vi "Slice Average calc.vi"(9 "end time (unix,ns)":u64, 10 "start time (unix,ns)":u64, 11 "Plot (unix)":T2) -> (2 "slice average":T1, 3 "Plot (unix)":T2)   [LabVIEW 2021, in "RocketPlot.lvlib"]
uses:
  RocketPlot.lvlib
  TypeDefs/plot datapoint.ctl
  TypeDefs/Slice average.ctl
  aeb3b9b0-3d0b-48fb-8ca9-3c9e8c208765.vi
  43998882-4a9d-44ca-a800-b6f182c48d79.vi
  <userlib>/bjustice/Ring Buffer for Time Series Data Strict Accessor/SubVIs/Search for oldest time to keep.vi
  <userlib>/bjustice/Ring Buffer for Time Series Data Strict Accessor/SubVIs/Search for newest time to keep.vi
  <userlib>/bjustice/Ring Buffer for Time Series Data Strict Accessor/Unix time epoch/Unix_Epoch_in_Labview.vi
  <vilib>/Analysis/NI_AALBase.lvlib
  <vilib>/Analysis/NI_AALPro.lvlib
  <userlib>/bjustice/Ring Buffer for Time Series Data Strict Accessor/Ring Buffer Strict Accessor.lvlib
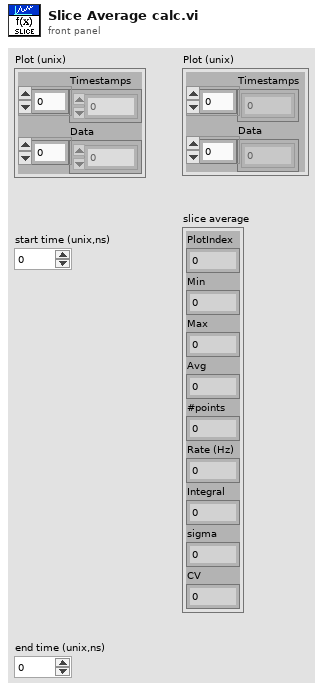
[diagram p1: front panel]
types:
  T1 = typedef "RocketPlot.lvlib/Slice average.ctl" = cluster{"PlotIndex":i32, "Min":dbl, "Max":dbl, "Avg":dbl, "#points":u32, "Rate (Hz)":dbl, "Integral":dbl, "sigma":dbl, "CV":dbl}
  T2 = typedef "RocketPlot.lvlib/plot datapoint.ctl" = cluster{"Timestamps":u64[], "Data":dbl[]}
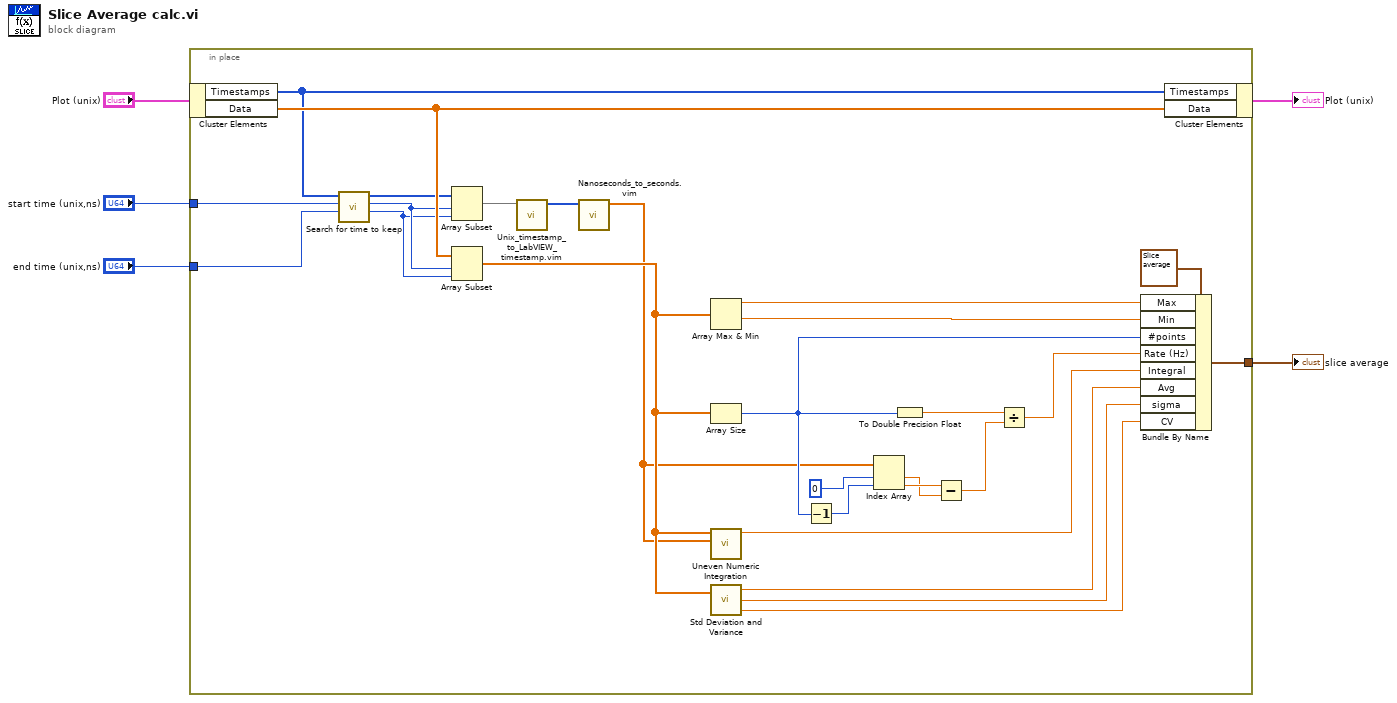
[diagram p0: block diagram]
diagram:
  n1 = in-place {
    in-place-border: "start time (unix,ns)" -> [w12]
    in-place-border: "end time (unix,ns)" -> [w11]
    in-place-border: [w15] -> w1
    n2 = in-place-cluster #1("Plot (unix)") -> ("Timestamps"=w14:u64[], "Data"=w16:dbl[])
    n3 = call <userlib>:"Search for time to keep.vi"("newest time to keep"=w11, "oldest time to keep"=w12, "timestamps (incrementing)"=w14) -> ("length"=w9:i32, "index"=w10:i32, "timestamps (dup)"=w13:u64[])  [unwired: 6 in]
    n4 = Array Subset(array=w13, index=w10, length=w9) -> (w8:u64[])
    n5 = Array Subset(array=w16, index=w10, length=w9) -> (w20:dbl[])
    n6 = call "Unix_timestamp_to_LabVIEW_timestamp.vim"("Unix timestamp (nanoseconds)"=w8) -> ("LabVIEW timestamp (nanoseconds)"=w7:u64[])  [unwired: 10 in]
    n7 = call "Nanoseconds_to_seconds.vim"("nanoseconds"=w7) -> ("seconds"=w6:dbl[])  [unwired: 10 in]
    n8 = Array Max & Min(array=w20) -> (max value=w31:dbl, min value=w30:dbl)  [unwired: 2 out]
    n9 = Array Size(array=w20) -> (size(s)=w24:i32)
    n10 = call <vilib>:"Uneven Numeric Integration.vi"("T"=w6, "X"=w20) -> ("result"=w27:dbl)  [unwired: 8 in, 1 out]
    n11 = call <vilib>:"Std Deviation and Variance.vi"("X"=w20) -> ("mean"=w19:dbl, "standard deviation"=w18:dbl, "variance"=w17:dbl)  [unwired: 1 in]
    n12 = Decrement(x=w24) -> (x-1=w29:i32)
    n13 = Index Array(array=w6, index #1=0 ("index"), index #2=w29) -> (element #1=w25:dbl, element #2=w26:dbl)
    n14 = To Double Precision Float(number=w24) -> (double precision float=w23:dbl)
    n15 = Subtract(x=w26, y=w25) -> (x-y=w22:dbl)
    n16 = Divide(x=w23, y=w22) -> (x/y=w21:dbl)
    n17 = Bundle By Name(cluster=T1 {"PlotIndex"=0, "Min"=0.0, "Max"=0.0, "Avg"=0.0, "#points"=0, "Rate (Hz)"=0.0, "Integral"=0.0, "sigma"=0.0, "CV"=0.0} ("Cluster"), "Max"=w31, "Min"=w30, "#points"=w24, "Rate (Hz)"=w21, "Integral"=w27, "Avg"=w19, "sigma"=w18, "CV"=w17) -> (w15:T1)
    n18 = in-place-cluster #1("Timestamps"=w14, "Data"=w16) -> (→"Plot (unix)":T2)
  }
  "slice average" <- w1
